vi "Set DIO Lines.vi"(8 "error in (no error)":errorcluster, 10 "DIO Lines":string[](array[string]), 11 "RIO Target in":refnum<class "RIO Target.lvclass">) -> (0 "error out":errorcluster, 3 "RIO Target out":refnum<class "RIO Target.lvclass">)   [LabVIEW 2014, in "RIO Target.lvclass"]
uses:
  RIO Target.lvclass
  RIO Target Configuration/RIO Target Configuration.lvclass
  RIO Target Configuration/RIO Target Configuration.lvclass/RIO Target Configuration.ctl
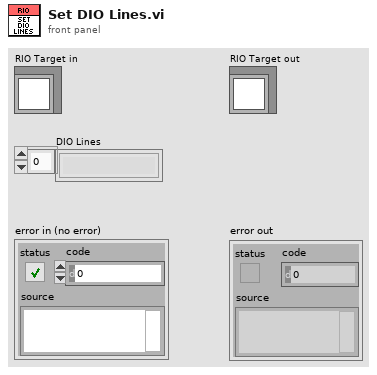
[diagram p1: front panel]
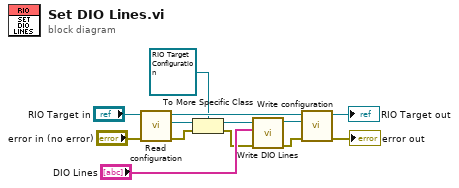
[diagram p0: block diagram]
diagram:
  n1 = call-dynamic "Read configuration.vi"("error in"="error in (no error)", "RIO Target in"="RIO Target in") -> ("error out"=w9:errorcluster, "configuration"=w7:refnum<class "NISE_CEF_serializable configuration.lvclass">, "RIO Target out"=w12:refnum<class "RIO Target.lvclass">)  [unwired: 7 in]
  n2 = To More Specific Class(target class=refnum<class "RIO Target Configuration.lvclass"> refnum ("RIO Target Configuration in"), reference=w7, error in=w9) -> (specific class reference=w6:refnum<class "RIO Target Configuration.lvclass">, error out=w3:errorcluster)
  n3 = call "Write DIO Lines.vi"("error in (no error)"=w3, "DIO Lines"="DIO Lines", "RIO Target Configuration in"=w6) -> ("error out"=w2:errorcluster, "RIO Target Configuration out"=w5:refnum<class "RIO Target Configuration.lvclass">)  [unwired: 7 in]
  n4 = call-dynamic "Write configuration.vi"("error in"=w2, "configuration"=w5, "RIO Target in"=w12) -> ("error out"=→"error out":errorcluster, "RIO Target out"=→"RIO Target out":refnum<class "RIO Target.lvclass">)  [unwired: 7 in]
